vi "Semantic_DialoguePyPl_Array_Msg.vi"(8 "error in (no error)":errorcluster caption="错误输入（无错误）", 10 "值(信号)":T1, 11 "States.lvlib:Voice.lvclass":refnum<class "Voice.lvclass">) -> (0 "error out":errorcluster caption="错误输出", 3 "Process State out":refnum<class "State Actor.lvclass">)   [LabVIEW 2014, in "States.lvlib" / "Voice.lvclass"]
uses:
  Voice.lvclass
  ctl/Semantic_Voice_Array.ctl
  <vilib>/NI/Actors/State Actor/State Actor/State Actor.lvclass
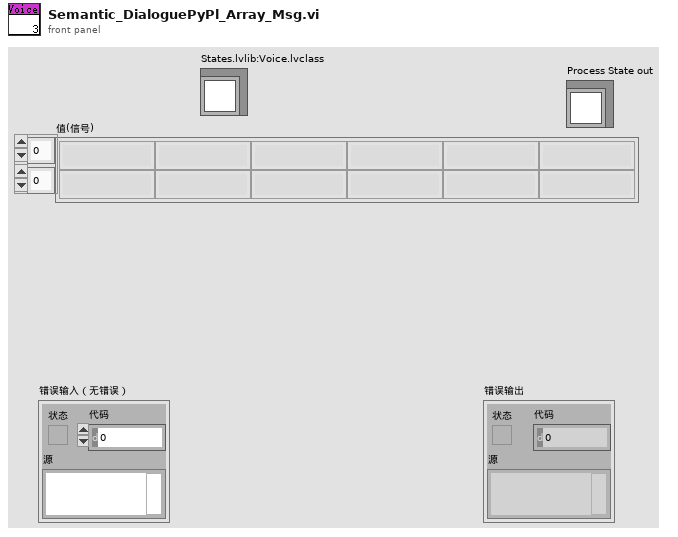
[diagram p1: front panel]
types:
  T1 = typedef "Semantic_Voice_Array.ctl" = string[][]
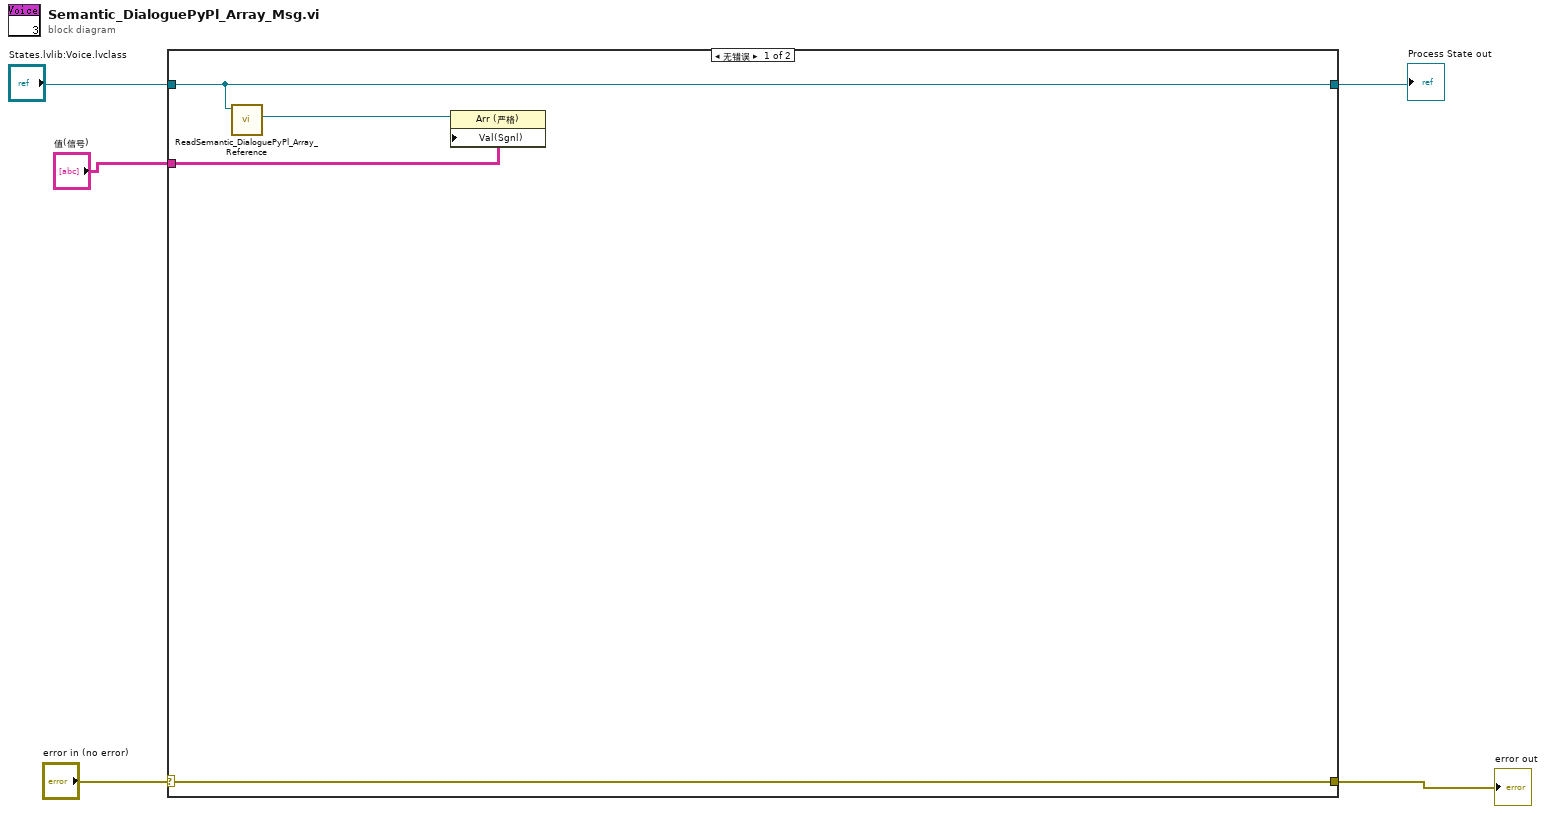
[diagram p0: block diagram]
diagram:
  n1 = case shown="无错误" "error in (no error)" {
    selector: "error in (no error)" -> [w9 w10]
    tunnel: [w9 w10] -> w4
    tunnel: [w7 w11] -> w2
    tunnel: "States.lvlib:Voice.lvclass" -> [w7 w11]
    tunnel: "值(信号)" -> [w8 _]
    frame No Error {
      n2 = call-dynamic "ReadSemantic_DialoguePyPl_Array_Reference.vi"("CoordinatorState输入"=w7) -> ("Semantic_DialoguePyPl_Array_Reference"=w6:refnum<vi>)  [unwired: 8 in, 2 out]
      n3 = property class="Arr (严格)"(reference=w6, "Val(Sgnl)"=w8) -> ()  [unwired: 1 in, 2 out]
    }
    frame Error {
    }
  }
  "error out" <- w4
  "Process State out" <- w2
